vi "Template Immediate.vi"(7 "Description":string, 8 "Command Info In":T1, 10 "Zeptrix":bool) -> (0 "Command Info Out":T1)   [LabVIEW 2020]
doc: "This template is useful for immediate subsystem actions that do not need deadband filtering\n\nBe sure to right-click and select New from Template and save with a new command name."
uses:
  <vilib>/Rock Robotics/WPI/Framework/Command Status Info.ctl
  <vilib>/Rock Robotics/WPI/Framework/Completion Status.ctl
  <vilib>/Rock Robotics/WPI/Framework/Completion Notifier.ctl
  Implementation/Climb Operations.ctl
  Implementation/Climb Setpoints.ctl
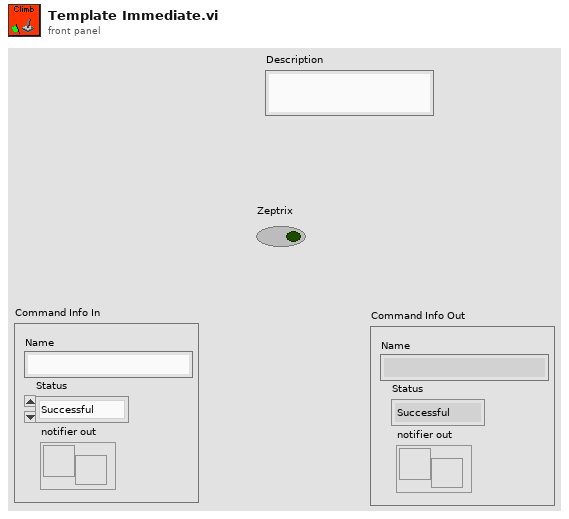
[diagram p1: front panel]
types:
  T1 = typedef "Command Status Info.ctl" = cluster{"Name":string, "Status":T2, "notifier out":T3}
  T2 = typedef "Completion Status.ctl" = enum16{"Successful", "Aborted", "Incomplete"}
  T3 = typedef "Completion Notifier.ctl" = refnum<notifier>
  T4 = typedef "Climb Operations.ctl" = enum16{"Reserve", "Read Current", "Immediate"}
  T5 = typedef "Climb Setpoints.ctl" = cluster{"Operation":T4, "Duration":dbl, "activated":bool}
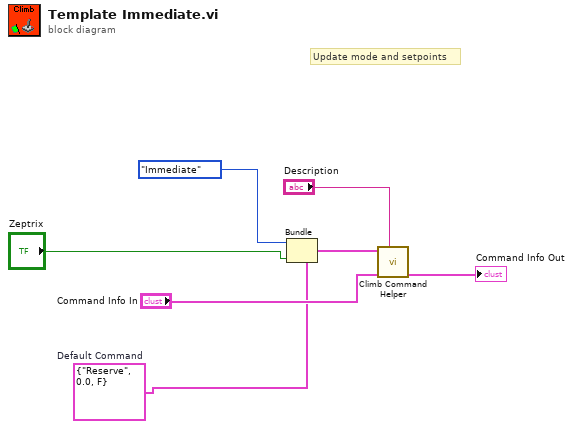
[diagram p0: block diagram]
diagram:
  w2 = T5 {"Operation"=enum."Reserve", "Duration"=0.0, "activated"=FALSE}  # Default Command
  # "Update mode and setpoints"
  n1 = Bundle(cluster=w2, "Operation"=Climb_Operations."Immediate", "activated"="Zeptrix") -> (w4:T5)  [unwired: 1 in]
  n2 = call "Climb Command Helper.vi"("Description"="Description", "Command Info In"="Command Info In", "SubSystem Data"=w4) -> ("Command Info Out"=→"Command Info Out":T1)  [unwired: 6 in, 2 out]
